vi "Play DMX Sound.vi"(8 "error in (no error)":errorcluster, 10 "Original Frq":u16=11025, 11 "Frequencies IN":u8[](array[numeric])=array[13815 elements]) -> (0 "error out":errorcluster)   [LabVIEW 2017]
uses:
  <vilib>/sound2/lvsound2.llb/Sampling Mode.ctl
  <vilib>/sound2/lvsound2.llb/Sound Data Format.ctl
  <vilib>/sound2/lvsound2.llb/Sound Output Write (DBL).vi
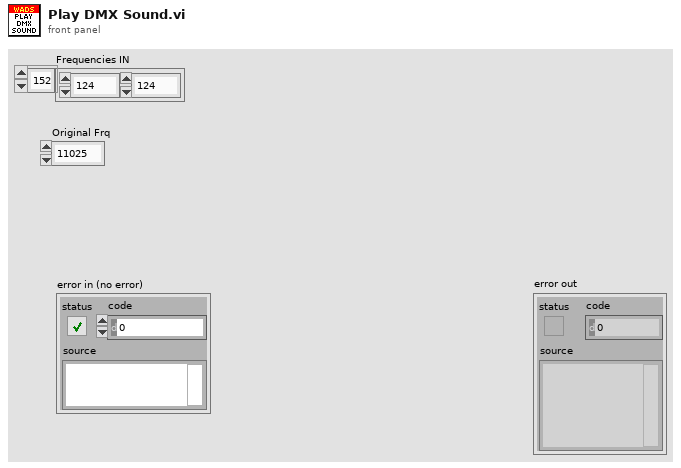
[diagram p1: front panel]
types:
  T1 = typedef "Sound Data Format.ctl" = cluster{"sample rate (S/s)":dbl, "number of channels":i32, "bits per sample":i32}
  T2 = typedef "Sampling Mode.ctl" = i32
  T3 = typedef "Sound Output Task ID.ctl" = u32
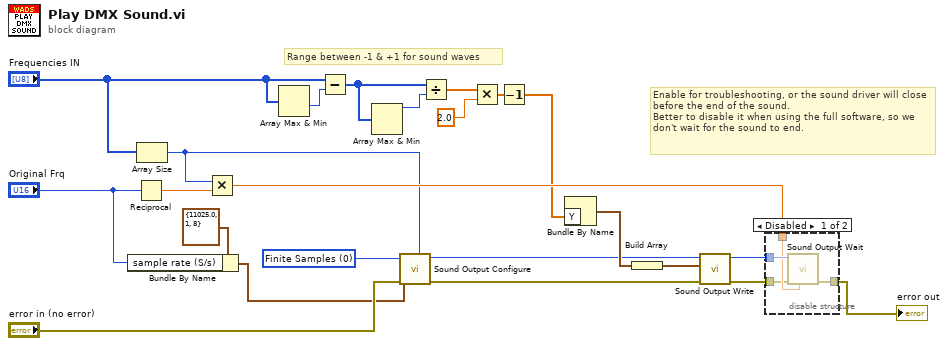
[diagram p0: block diagram]
diagram:
  w23 = T2 0 items=["Finite Samples", "Continuous Samples"] ("sample mode")
  # "Enable for troubleshooting, or the sound driver will close before the end of the sound.\nBetter to disable it when using the full software, so we don't wait for the sound to end."
  # "Range between -1 & +1 for sound waves"
  n1 = Bundle By Name(cluster=T1 {"sample rate (S/s)"=11025.0, "number of channels"=1, "bits per sample"=8} ("sound format"), "sample rate (S/s)"="Original Frq") -> (w12:T1)
  n2 = Reciprocal(x="Original Frq") -> (1/x=w19:dbl)
  n3 = Array Size(array="Frequencies IN") -> (size(s)=w11:i32)
  n4 = Multiply(x=w11, y=w19) -> (x*y=w17:dbl)
  n5 = Array Max & Min(array="Frequencies IN") -> (min value=w5:u8)  [unwired: 3 out]
  n6 = Subtract(x="Frequencies IN", y=w5) -> (x-y=w4:u8[])
  n7 = Array Max & Min(array=w4) -> (max value=w8:u8)  [unwired: 3 out]
  n8 = call <vilib>:"Sound Output Configure.vi"("number of samples/ch"=w11, "sample mode"=w23, "error in (no error)"="error in (no error)", "sound format"=w12) -> ("error out"=w2:errorcluster, "task ID"=w3:T3)  [unwired: 6 in]
  n9 = Divide(x=w4, y=w8) -> (x/y=w9:dbl[])
  n10 = Multiply(x=w9, y=2.0 ("Compression parameter")) -> (x*y=w7:dbl[])
  n11 = Decrement(x=w7) -> (x-1=w6:dbl[])
  n12 = Bundle By Name("Y"=w6) -> (w22:waveform(dbl))  [unwired: 1 in]
  n13 = Build Array(w22) -> (w21:waveform(dbl)[])
  n14 = call-poly <vilib>:"Sound Output Write.vi"("error in (no error)"=w2, "data"=w21, "task ID"=w3) -> ("error out"=w16:errorcluster, "task ID out"=w18:T3)  [unwired: 7 in]
  n15 = disable-structure shown="Disabled" {
    disable-tunnel: w18 -> [w27 _]
    disable-tunnel: w17 -> [w26 _]
    disable-tunnel: w16 -> [w25 w28]
    disable-tunnel: [w24 w28] -> w15
    frame Disabled {
      n16 = call <vilib>:"Sound Output Wait.vi"("timeout (sec)"=w26, "error in (no error)"=w25, "task ID"=w27) -> ("error out"=w24:errorcluster)  [unwired: 7 in, 1 out]
    }
    frame Enabled {
    }
  }
  "error out" <- w15
